vi "lesker(SubVI).vi"(11 "stop":bool) -> (3 "Pressure (Torr)":dbl)   [LabVIEW 2012]
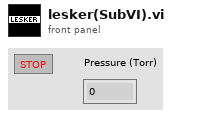
[diagram p1: front panel]
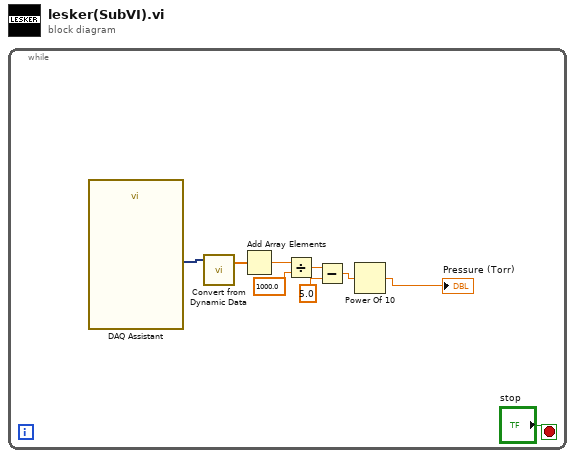
[diagram p0: block diagram]
diagram:
  n1 = while {
    stop <- "stop" stop-if-true
    n2 = call "DAQ Assistant"() -> ("data"=w3:dynamicdata)  [unwired: 17 in, 2 out]
    n3 = call "Convert from Dynamic Data"("Dynamic Data Type"=w3) -> ("Array"=w8:dbl[])  [unwired: 3 in]
    n4 = Add Array Elements(numeric array=w8) -> (sum=w7:dbl)
    n5 = Divide(x=w7, y=1000.0) -> (x/y=w5:dbl)
    n6 = Subtract(x=w5, y=5.0) -> (x-y=w4:dbl)
    n7 = Power Of 10(x=w4) -> (10^x=→"Pressure (Torr)":dbl)
  }
